vi "UTF8 Encoding to UTF16 Encoding.vi"(6 "Big Endian?":bool, 8 "error in (no error)":errorcluster, 9 "UTF-8 String":string) -> (0 "error out":errorcluster, 1 "UTF-16 String":string)   [LabVIEW 2011]
doc: "Converts teh UTF-8 Encoded string to UTF-16LE encoded string."
uses:
  Numeric/Conversion/To [U8] BigEndian.llb/[U16] To [U8] BigEndian.vi
  Numeric/Conversion/To [U8].llb/[U16] To [U8].vi
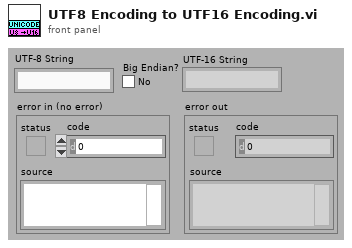
[diagram p1: front panel]
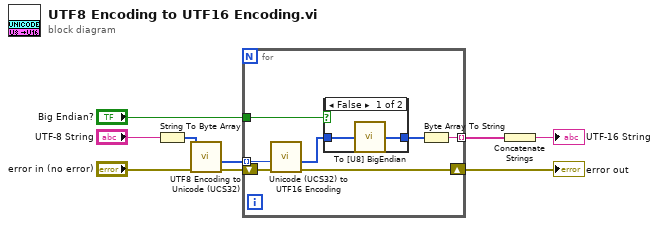
[diagram p0: block diagram]
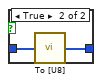
[diagram p2: hidden frame]
diagram:
  n1 = String To Byte Array(string="UTF-8 String") -> (unsigned byte array=w4:u8[])
  n2 = call "UTF8 Encoding to Unicode (UCS32).vi"("error in"="error in (no error)", "[UTF-8]"=w4) -> ("error out"=w1:errorcluster, "[UCS 32]"=w2:u32[])  [unwired: 7 in, 1 out]
  n3 = for {
    tunnel: [w14] -> w9 mode=indexing
    shift-right: [w10] -> w6
    shift-left: w1 -> [w12]
    tunnel: "Big Endian?" -> [w15]
    tunnel: w2 -> [w13] mode=indexing
    n4 = call "Unicode (UCS32) to UTF16 Encoding.vi"("error in"=w12, "[UCS 32]"=w13) -> ("error out"=w10:errorcluster, "[UTF-16]"=w11:u16[])  [unwired: 8 in]
    n5 = case shown="False" w15 {
      tunnel: [w18 w19] -> w16
      tunnel: w11 -> [w17 w20]
      frame False {
        n6 = call-poly "To [U8] BigEndian.vi"("U16 Array"=w17) -> ("U8 Array"=w18:u8[])  [unwired: 4 in]
      }
      frame True {
        n7 = call-poly "To [U8].vi"("U16 Array"=w20) -> ("U8 Array"=w19:u8[])  [unwired: 4 in]
      }
    }
    n8 = Byte Array To String(unsigned byte array=w16) -> (string=w14:string)
  }
  "error out" <- w6
  n9 = Concatenate Strings(w9) -> (→"UTF-16 String":string)
